vi "face_hand.vi"() -> ()   [LabVIEW 2025]
uses:
  <vilib>/Platform/TimedLoop/XDataNode/timing_clust.ctl
  <vilib>/Platform/TimedLoop/XDataNode/nitl_modes.ctl
  <vilib>/Platform/TimedLoop/XDataNode/wakeup.ctl
  <vilib>/platform/TimedLoop/XDataNode/XDataNode.xnode
  <vilib>/Platform/TimedLoop/XDataNode/XDNodeRunTimeDep.lvlib
panel:
  out "错误输出":errorcluster
  out "路径":path
  out "文本":string
  out "上次修改":timestamp
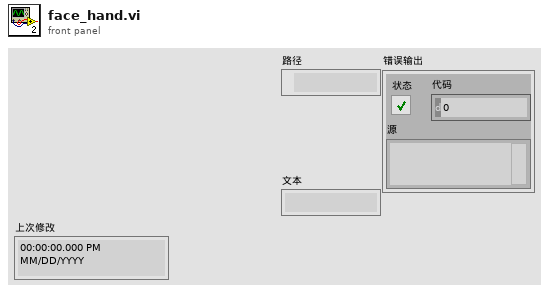
[diagram p1: front panel]
types:
  T1 = typedef "XDNodeRunTimeDep.lvlib/timing_clust.ctl" = cluster{"Expected End [f-1]":u64, "Actual End [f-1]":u64, "Finished Late? [f-1]":bool, "Expected End [i-1]":u64, "Actual End [i-1]":u64, "Finished Late? [i-1]":bool, "Expected Start [i]":u64, "Actual Start [i]":u64, "Expected Start [f]":u64, "Actual Start [f]":u64, "Source Name":string, "Structure Name":string, "Period":i64, "Deadline":i64, "Offset":i64, "Start":i64, "Priority":i32, "Timeout":i32, "Mode":T2, "Wakeup Reason":T3, "Error":errorcluster, "Source Type":string, "Secondary Source Type":string, "Global End Time":u64, "Global Start Time":u64, "Frame Duration":u64, "Iteration Duration":u64, "Assigned CPU":i32, "I/O Scan Engine Mode":u32}
  T2 = typedef "XDNodeRunTimeDep.lvlib/nitl_modes.ctl" = enum32{"No Change", "Process missed periods, maintain original phase", "Discard missed periods, maintain original phase", "Process missed periods, ignore original phase", "Discard missed periods, ignore original phase"}
  T3 = typedef "XDNodeRunTimeDep.lvlib/wakeup.ctl" = enum32{"Normal", "Aborted", "Asynchronous wakeup", "Timing source error", "Timed loop error", "Timeout"}
  T4 = enum16{"open", "replace", "create", "open or create", "replace or create", "replace or create with confirmation"}
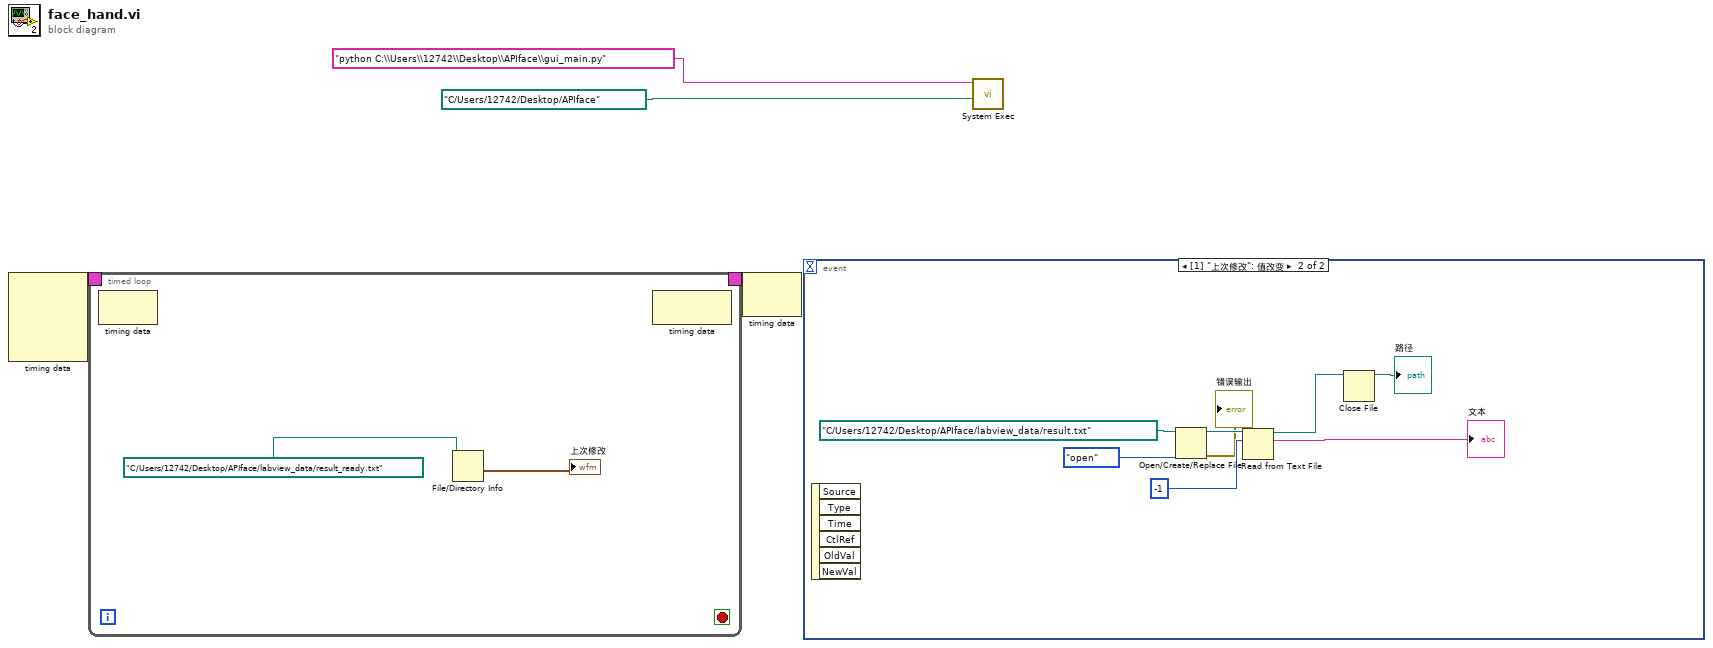
[diagram p0: block diagram]
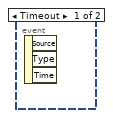
[diagram p2: hidden frame]
diagram:
  n1 = node-c288() -> (w4:T1)  [unwired: 4 in]
  n2 = timed-loop {
    timing: w4 -> [_]
    timing-out: [_] -> w3
    stop <- _ stop-if-true
    n3 = node-c288() -> ()  [unwired: 1 in, 1 out]
    n4 = File/Directory Info(path=path "C:/Users/12742/Desktop/APIface/labview_data/result_ready.txt" ("路径")) -> (last mod=→"上次修改":timestamp)  [unwired: 1 in, 6 out]
    n5 = node-c288() -> ()  [unwired: 1 in, 1 out]
  }
  n6 = node-c288(w3) -> ()  [unwired: 1 out]
  n7 = event shown="[1] \"上次修改\": 值改变" {
    selector: _ -> [_ _]
    dyn-events: _ -> [_ _]
    timeout: _ -> [_ _]
    event Timeout {
      n8 = event-data() -> ()  [unwired: 1 in, 3 out]
    }
    event "上次修改": Value Change {
      n9 = event-data() -> ()  [unwired: 1 in, 6 out]
      n10 = Open/Create/Replace File(file path (use dialog)=path "C:/Users/12742/Desktop/APIface/labview_data/result.txt" ("文件路径（使用对话框）"), operation (0:open)=T4."open" ("操作(0:open)")) -> (refnum out=w13:refnum<file>, error out=→"错误输出":errorcluster)  [unwired: 4 in, 1 out]
      n11 = Read from Text File(file (use dialog)=w13, count=-1 ("计数")) -> (refnum out=w12:refnum<file>, text=→"文本":string)  [unwired: 2 in, 2 out]
      n12 = Close File(refnum=w12) -> (path=→"路径":path)  [unwired: 1 in, 1 out]
    }
  }
  n13 = call <vilib>:"System Exec.vi"("working directory"=path "C:/Users/12742/Desktop/APIface", "command line"="python C:\\Users\\12742\\Desktop\\APIface\\gui_main.py") -> ()  [unwired: 6 in, 4 out]
